vi "Get Attribute BOOL.vi"(8 "error in":errorcluster, 10 "Attribute":string, 11 "Config from EXCEL in":refnum<class "Config from EXCEL.lvclass">) -> (0 "error out":errorcluster, 2 "Value":bool, 3 "Config from EXCEL out":refnum<class "Config from EXCEL.lvclass">)   [LabVIEW 2024, in "Config from EXCEL.lvclass"]
uses:
  Config from EXCEL.lvclass
  Config from EXCEL.lvclass/Config from EXCEL.ctl
  Open-Xml-LabVIEW/Source/Open Xml.lvlib
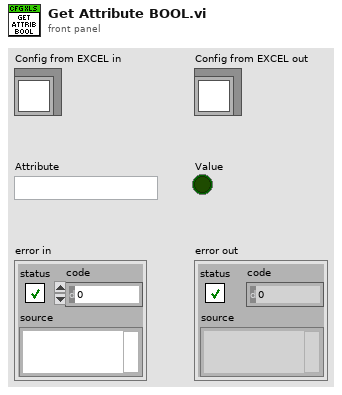
[diagram p1: front panel]
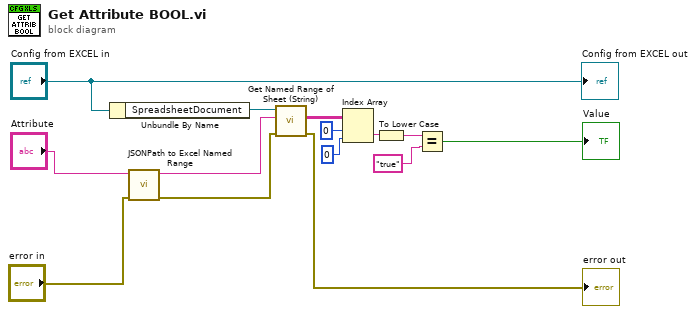
[diagram p0: block diagram]
diagram:
  n1 = Unbundle By Name("Config from EXCEL in") -> ("SpreadsheetDocument"=w14:refnum<k24>)
  n2 = call "JSONPath to Excel Named Range.vi"("error in"="error in", "JSONPath"="Attribute") -> ("error out"=w9:errorcluster, "Named Range"=w13:string)  [unwired: 8 in]
  n3 = call "Get Named Range of Sheet (String).vi"("error in"=w9, "Named Range Identifier"=w13, "SpreadsheetDocument"=w14) -> ("error out"=→"error out":errorcluster, "Cells"=w12:string[][])  [unwired: 6 in, 1 out]
  n4 = Index Array(array=w12, index (row)=0, index (col)=0) -> (element=w4:string)
  n5 = To Lower Case(string=w4) -> (all lower case string=w3:string)
  n6 = Equal?(x=w3, y="true") -> (x = y?=→"Value":bool)
  "Config from EXCEL out" <- "Config from EXCEL in"
